vi "Data Analysis.vi"(1 "Data Collection Mode":enum32{"Reference", "Sample"}(radio), 9 "Cluster":T4, 11 "Experimental Parameters":T1={"Correction Factor"=0.0, "Data Interval (s)"=0.0, "Number of Data Points"=0.0, "Incident Angle (Degrees)"=0.0, "Refractive Index (Rare)"=0.0, "Refractive Index (Dense)"=0.0, "PMT Bias Voltage (V)"=0.0, "Laser Wavelength (nm)"=0.0, "Preamplifier Output Gain (uA/V)"=0.0, "PEM Monitoring Frequency"=1} {"PEM Monitoring Frequency" min=1 max=2 step=1}) -> (4 "Reference Analysis":T5, 6 "Sample Analysis":T2, 10 "Reference Averages":T3, 15 "Sample Averages":T3)   [LabVIEW 2017, in "LD Reading.lvclass"]
uses:
  LD Reading.lvclass
  Reference Channel Intensities.ctl
  Average Data.ctl
  Sample Channel Intensities.ctl
  Experimental Parameters.ctl
  <vilib>/Analysis/baseanly.llb/Mean (DBL).vi
  <vilib>/Analysis/NI_AALBase.lvlib
panel:
  # "Data Collection Parameters"
  # "System Settings"
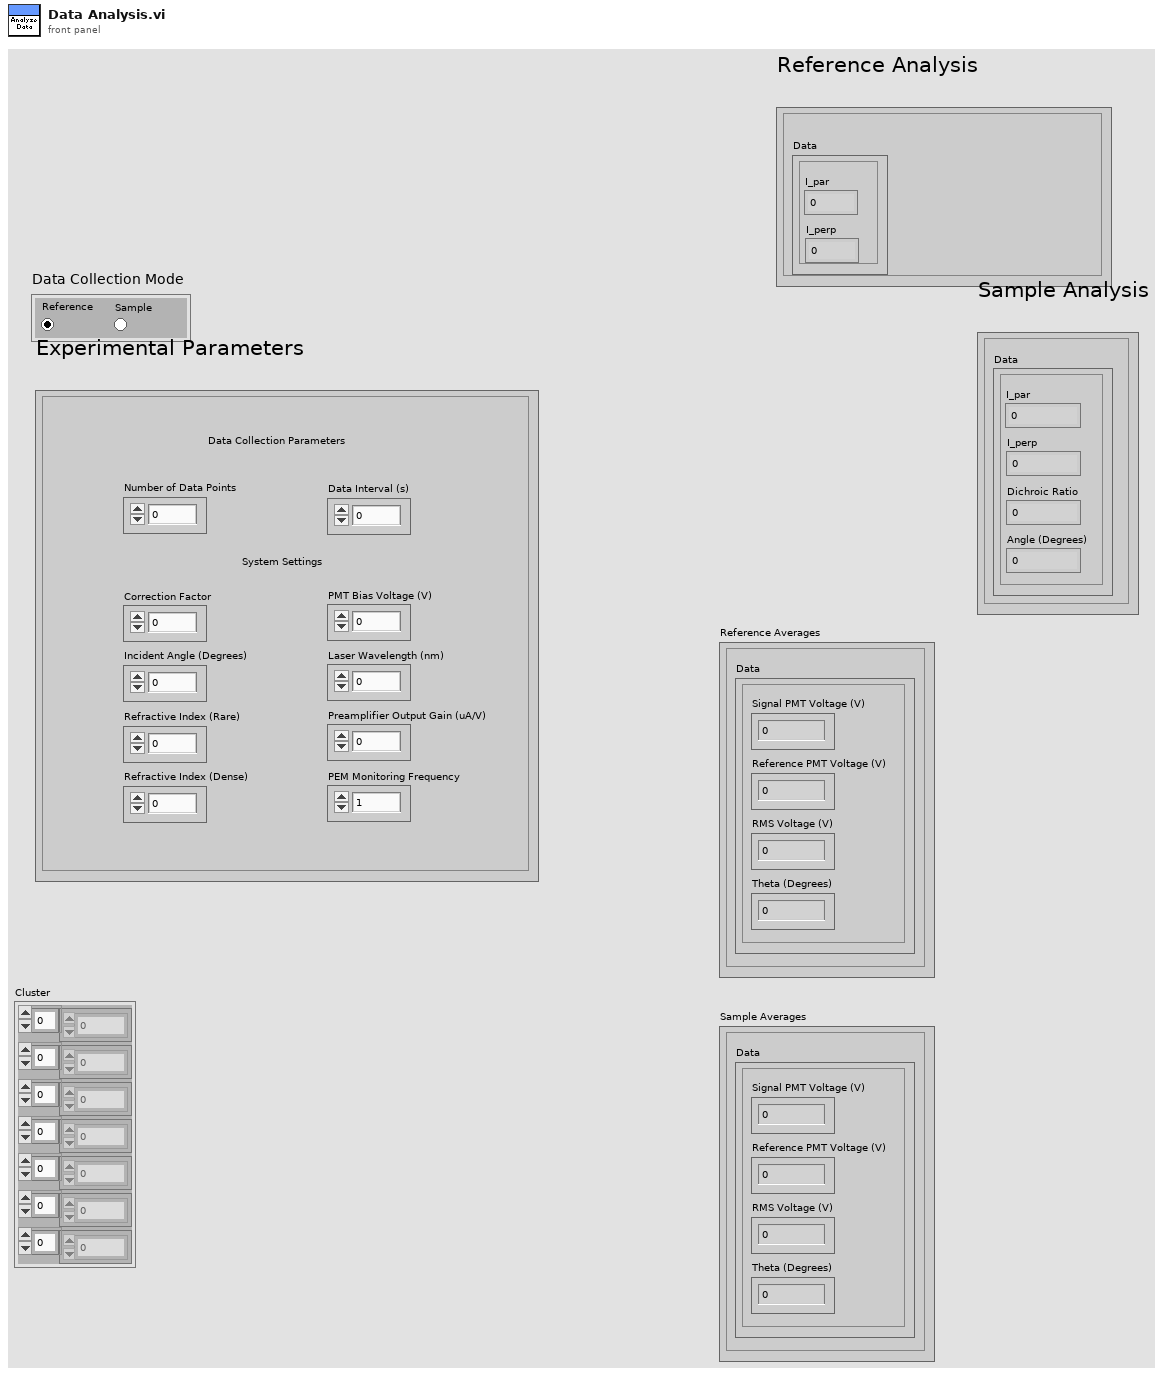
[diagram p1: front panel]
types:
  T1 = typedef "Experimental Parameters.ctl" = cluster{"Correction Factor":dbl, "Data Interval (s)":dbl, "Number of Data Points":dbl, "Incident Angle (Degrees)":dbl, "Refractive Index (Rare)":dbl, "Refractive Index (Dense)":dbl, "PMT Bias Voltage (V)":dbl, "Laser Wavelength (nm)":dbl, "Preamplifier Output Gain (uA/V)":dbl, "PEM Monitoring Frequency":u8}
  T2 = typedef "Sample Channel Intensities.ctl" = cluster{"Data":cluster{"I_par":dbl, "I_perp":dbl, "Dichroic Ratio":dbl, "Angle (Degrees)":dbl}}
  T3 = typedef "Average Data.ctl" = cluster{"Data":cluster{"Signal PMT Voltage (V)":dbl, "Reference PMT Voltage (V)":dbl, "RMS Voltage (V)":dbl, "Theta (Degrees)":dbl}}
  T4 = cluster{dbl[], dbl[], dbl[], dbl[], dbl[], dbl[], dbl[]}
  T5 = typedef "Reference Channel Intensities.ctl" = cluster{"Data":cluster{"I_par":dbl, "I_perp":dbl}}
  T6 = cluster{"Signal PMT Voltage (V)":dbl, "Reference PMT Voltage (V)":dbl, "RMS Voltage (V)":dbl, "Theta (Degrees)":dbl}
  T7 = cluster{"I_par":dbl, "I_perp":dbl, "Dichroic Ratio":dbl, "Angle (Degrees)":dbl}
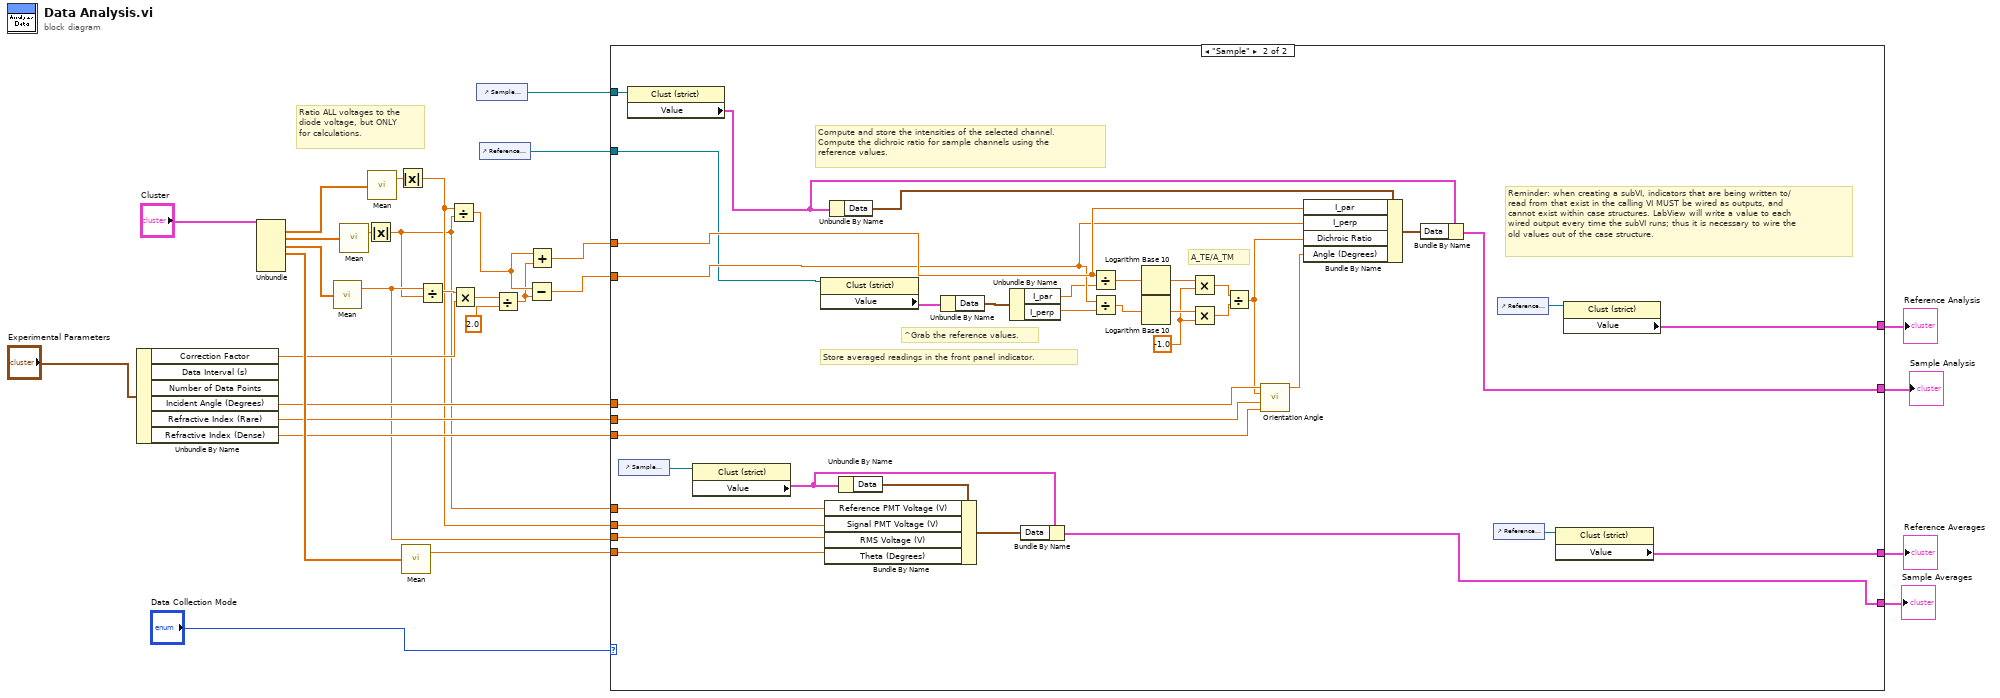
[diagram p0: block diagram]
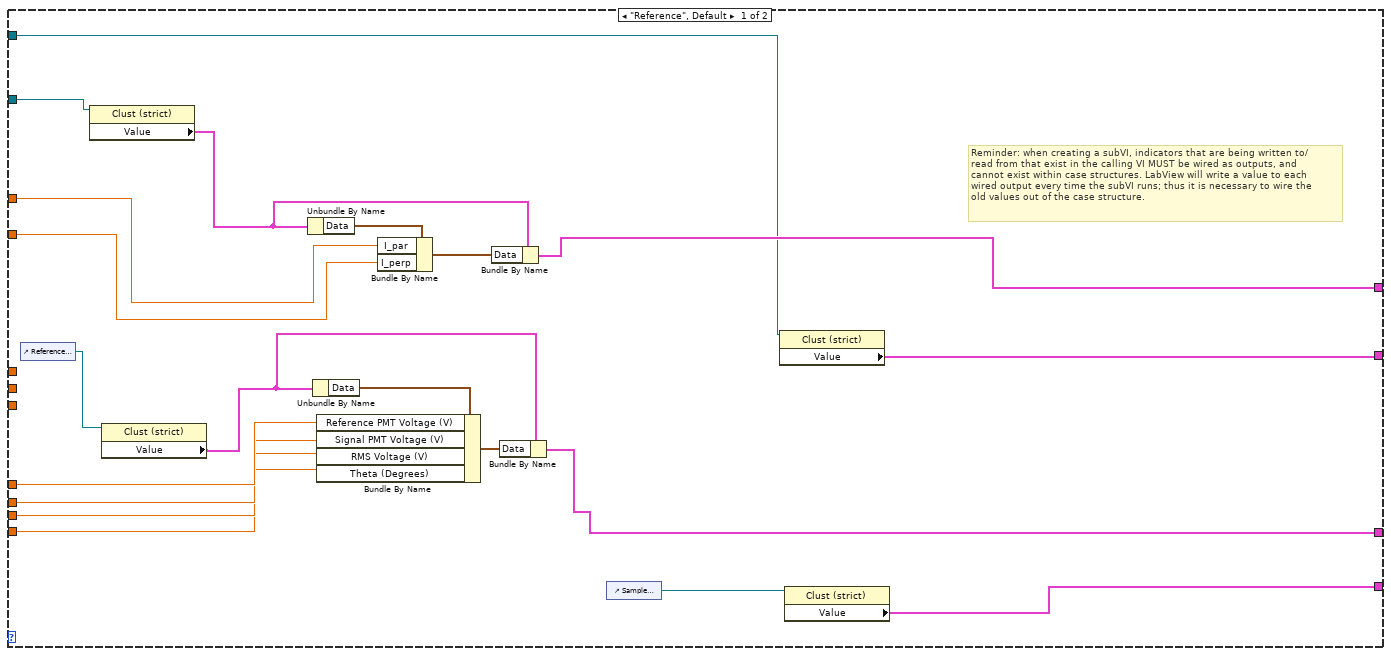
[diagram p2: hidden frame]
diagram:
  # "Ratio ALL voltages to the \ndiode voltage, but ONLY \nfor calculations."
  n1 = Unbundle By Name("Experimental Parameters") -> ("Correction Factor"=w14:dbl, "Incident Angle (Degrees)"=w13:dbl, "Refractive Index (Rare)"=w12:dbl, "Refractive Index (Dense)"=w11:dbl)  [unwired: 2 out]
  n2 = Unbundle("Cluster") -> (w29:dbl[], w28:dbl[], w30:dbl[], w19:dbl[])  [unwired: 3 out]
  n3 = call-poly <vilib>:"Mean.vi"("X"=w30) -> ("mean"=w7:dbl)  [unwired: 1 out]
  n4 = call-poly <vilib>:"Mean.vi"("X"=w28) -> ("mean"=w8:dbl)  [unwired: 1 out]
  n5 = Absolute Value(x=w8) -> (abs(x)=w1:dbl)
  n6 = call-poly <vilib>:"Mean.vi"("X"=w29) -> ("mean"=w10:dbl)  [unwired: 1 out]
  n7 = Absolute Value(x=w10) -> (abs(x)=w2:dbl)
  n8 = call-poly <vilib>:"Mean.vi"("X"=w19) -> ("mean"=w18:dbl)  [unwired: 1 out]
  n9 = Divide(x=w7, y=w1) -> (x/y=w9:dbl)
  n10 = Divide(x=w2, y=w1) -> (x/y=w26:dbl)
  n11 = Multiply(x=w9, y=w14) -> (x*y=w21:dbl)
  n12 = control-ref of="Sample Analysis"() -> (w17:refnum<vi>)
  n13 = control-ref of="Reference Analysis"() -> (w16:refnum<vi>)
  n14 = Divide(x=w21, y=2.0) -> (x/y=w23:dbl)
  n15 = Subtract(x=w26, y=w23) -> (x-y=w25:dbl)
  n16 = Add(x=w26, y=w23) -> (x+y=w24:dbl)
  n17 = case shown="\"Sample\"" "Data Collection Mode" {
    tunnel: w24 -> [w50 w87]
    tunnel: w25 -> [w49 w86]
    tunnel: [w46 w68] -> w5
    tunnel: [w47 w84] -> w6
    tunnel: [w44 w75] -> w3
    tunnel: w1 -> [w41 w79]
    tunnel: w2 -> [w40 w78]
    tunnel: w7 -> [w39 w77]
    tunnel: w18 -> [w38 w76]
    tunnel: [w37 w82] -> w4
    tunnel: w17 -> [w35 w73]
    tunnel: w16 -> [w36 w72]
    tunnel: w13 -> [_ w71]
    tunnel: w12 -> [_ w70]
    tunnel: w11 -> [_ w69]
    frame "Reference", Default {
      # "Reminder: when creating a subVI, indicators that are being written to/\nread from that exist in the calling VI MUST be wired as outputs, and \ncannot exist within case structures. LabView will write a value to each \nwired output every time the subVI runs; thus it is necessary to wire the \nold values out of the case structure."
      n18 = control-ref of="Reference Averages"() -> (w43:refnum<vi>)
      n19 = property class="Clust (strict)"(reference=w36) -> ("Value"=w48:T5)  [unwired: 1 in, 2 out]
      n20 = property class="Clust (strict)"(reference=w43) -> ("Value"=w42:T3)  [unwired: 1 in, 2 out]
      n21 = Unbundle By Name(w48) -> ("Data"=w33:cluster{"I_par":dbl, "I_perp":dbl})
      n22 = Unbundle By Name(w42) -> ("Data"=w32:T6)
      n23 = Bundle By Name(cluster=w32, "Reference PMT Voltage (V)"=w41, "Signal PMT Voltage (V)"=w40, "RMS Voltage (V)"=w39, "Theta (Degrees)"=w38) -> (w31:T6)
      n24 = Bundle By Name(cluster=w33, "I_par"=w50, "I_perp"=w49) -> (w34:cluster{"I_par":dbl, "I_perp":dbl})
      n25 = Bundle By Name(cluster=w48, "Data"=w34) -> (w47:T5)
      n26 = Bundle By Name(cluster=w42, "Data"=w31) -> (w37:T3)
      n27 = control-ref of="Sample Averages"() -> (w45:refnum<vi>)
      n28 = property class="Clust (strict)"(reference=w35) -> ("Value"=w46:T2)  [unwired: 1 in, 2 out]
      n29 = property class="Clust (strict)"(reference=w45) -> ("Value"=w44:T3)  [unwired: 1 in, 2 out]
    }
    frame "Sample" {
      w59 = -1.0
      # "A_TE/A_TM"
      # "^Grab the reference values."
      # "Store averaged readings in the front panel indicator."
      # "Compute and store the intensities of the selected channel. \nCompute the dichroic ratio for sample channels using the \nreference values."
      # "Reminder: when creating a subVI, indicators that are being written to/\nread from that exist in the calling VI MUST be wired as outputs, and \ncannot exist within case structures. LabView will write a value to each \nwired output every time the subVI runs; thus it is necessary to wire the \nold values out of the case structure."
      n30 = control-ref of="Sample Averages"() -> (w81:refnum<vi>)
      n31 = property class="Clust (strict)"(reference=w73) -> ("Value"=w74:T2)  [unwired: 1 in, 2 out]
      n32 = property class="Clust (strict)"(reference=w81) -> ("Value"=w80:T3)  [unwired: 1 in, 2 out]
      n33 = property class="Clust (strict)"(reference=w72) -> ("Value"=w67:T5)  [unwired: 1 in, 2 out]
      n34 = Unbundle By Name(w74) -> ("Data"=w56:T7)
      n35 = Unbundle By Name(w80) -> ("Data"=w58:T6)
      n36 = Bundle By Name(cluster=w58, "Reference PMT Voltage (V)"=w79, "Signal PMT Voltage (V)"=w78, "RMS Voltage (V)"=w77, "Theta (Degrees)"=w76) -> (w57:T6)
      n37 = Unbundle By Name(w67) -> ("Data"=w66:cluster{"I_par":dbl, "I_perp":dbl})
      n38 = Unbundle By Name(w66) -> ("I_par"=w65:dbl, "I_perp"=w64:dbl)
      n39 = Bundle By Name(cluster=w80, "Data"=w57) -> (w75:T3)
      n40 = Divide(x=w87, y=w65) -> (x/y=w62:dbl)
      n41 = Divide(x=w86, y=w64) -> (x/y=w63:dbl)
      n42 = Logarithm Base 10(1:w62) -> (0:w60:dbl)
      n43 = Logarithm Base 10(1:w63) -> (0:w61:dbl)
      n44 = Multiply(x=w60, y=w59) -> (x*y=w51:dbl)
      n45 = Multiply(x=w61, y=w59) -> (x*y=w52:dbl)
      n46 = Divide(x=w51, y=w52) -> (x/y=w54:dbl)
      n47 = call "Orientation Angle.vi"("Refractive Index (Dense)"=w69, "Refractive Index (Rare)"=w70, "Dichroic Ratio"=w54, "Incident Angle (Degrees)"=w71) -> ("Orientation Angle (Degrees)"=w55:dbl)  [unwired: 7 in]
      n48 = Bundle By Name(cluster=w56, "I_par"=w87, "I_perp"=w86, "Dichroic Ratio"=w54, "Angle (Degrees)"=w55) -> (w53:T7)
      n49 = Bundle By Name(cluster=w74, "Data"=w53) -> (w68:T2)
      n50 = control-ref of="Reference Averages"() -> (w83:refnum<vi>)
      n51 = control-ref of="Reference Analysis"() -> (w85:refnum<vi>)
      n52 = property class="Clust (strict)"(reference=w83) -> ("Value"=w82:T3)  [unwired: 1 in, 2 out]
      n53 = property class="Clust (strict)"(reference=w85) -> ("Value"=w84:T5)  [unwired: 1 in, 2 out]
    }
  }
  "Reference Analysis" <- w6
  "Reference Averages" <- w4
  "Sample Averages" <- w3
  "Sample Analysis" <- w5
